vi "Print Buffer.vi"(0 "VISA resource name":refnum<visa-resource-name>, 1 "Start Index (1)":u32=1, 2 "Timeout (2000 ms)":u32=2000, 3 "End Index (1)":u32=1, 9 "Buffer Name(s)":string, 11 "error in (no error)":errorcluster, 12 "Byte Count (1024)":u32=1024) -> (4 "VISA resource name out":refnum<visa-resource-name>, 6 "Return Count":u32, 10 "Buffer Data":string, 14 "Command String":string, 15 "error out":errorcluster)   [LabVIEW 2009, in "Keithley 2600 Series.lvlib"]
doc: "This VI instructs the instrument to print the contents of the reading buffers and tables defined by <b>Buffer Name(s)</b> to the instrument data output queue.\n\n<b>Functions and Attributes Used</b>\nprintbuffer(start_index, end_index, st_1, ...)"
uses:
  <instrlib>/Keithley 2600 Series/Keithley 2600 Series.lvlib
  <instrlib>/Keithley 2600 Series/Private/GlobalVariables.vi
panel:
  # "(c) 2008 Keithley Instruments, Inc.  ALL RIGHTS RESERVED."
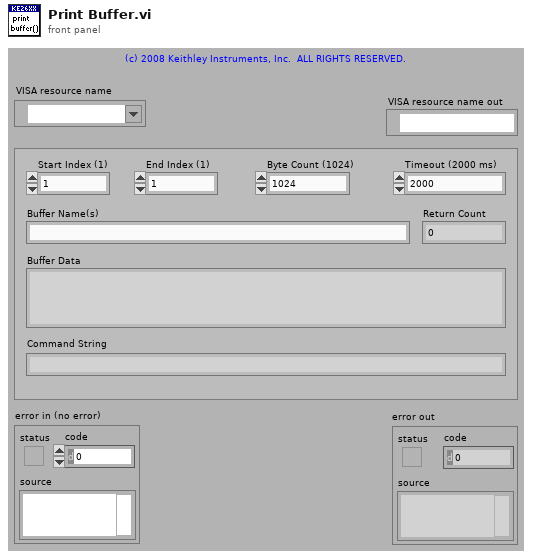
[diagram p1: front panel]
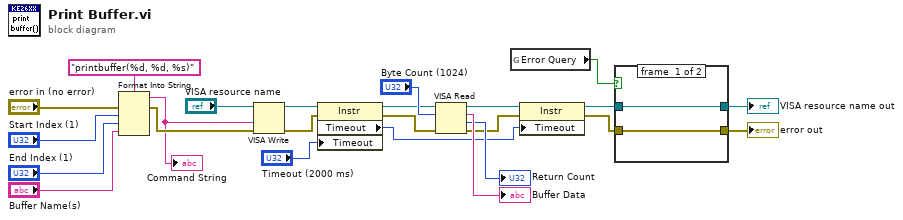
[diagram p0: block diagram]
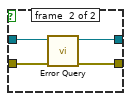
[diagram p2: hidden frame]
diagram:
  n1 = Format Into String(format string="printbuffer(%d, %d, %s)", error in="error in (no error)", "Start Index (1)", "End Index (1)", "Buffer Name(s)") -> (resulting string=w16:string, error out=w17:errorcluster)  [unwired: 1 in]
  "Command String" <- w16
  n2 = VISA Write(VISA resource name="VISA resource name", write buffer=w16, error in (no error)=w17) -> (VISA resource name out=w8:refnum<visa-resource-name>, error out=w7:errorcluster)  [unwired: 1 out]
  n3 = property class="Instr"(reference=w8, error in=w7, "Timeout"="Timeout (2000 ms)") -> (reference out=w10:refnum<visa-resource-name>, error out=w9:errorcluster, "Timeout"=w11:u32)
  n4 = VISA Read(VISA resource name=w10, byte count="Byte Count (1024)", error in (no error)=w9) -> (VISA resource name out=w13:refnum<visa-resource-name>, read buffer=→"Buffer Data":string, return count=→"Return Count":u32, error out=w12:errorcluster)
  n5 = global read "GlobalVariables.vi" "Error Query"() -> (w4:bool)
  n6 = property class="Instr"(reference=w13, error in=w12, "Timeout"=w11) -> (reference out=w5:refnum<visa-resource-name>, error out=w3:errorcluster)
  n7 = case shown="True" w4 {
    tunnel: w5 -> [w26 w30]
    tunnel: w3 -> [w25 w29]
    tunnel: [w26 w28] -> w1
    tunnel: [w25 w27] -> w2
    frame #0 {
    }
    frame #1 {
      n8 = call <instrlib>:"Error Query.vi"("error in (no error)"=w29, "VISA resource name"=w30) -> ("error out"=w27:errorcluster, "VISA resource name out"=w28:refnum<visa-resource-name>)  [unwired: 8 out]
    }
  }
  "error out" <- w2
  "VISA resource name out" <- w1
